vi "Unsubscribe Class Topic.vi"(7 "Close if last?":bool, 8 "error in (no error)":errorcluster, 10 "Receivers Enqueuer":refnum<class "Message Enqueuer.lvclass">, 11 "Topic":refnum<class>) -> (0 "error out":errorcluster)   [LabVIEW 2020, in "Actor Pub Sub Channels.lvlib"]
uses:
  Actor Pub Sub Channels.lvlib
  <vilib>/ActorFramework/Message Enqueuer/Message Enqueuer.lvclass
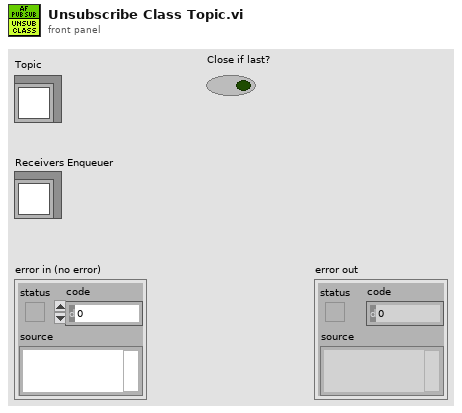
[diagram p1: front panel]
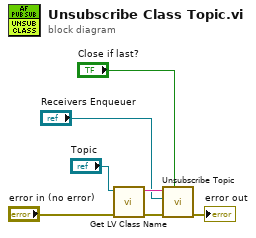
[diagram p0: block diagram]
diagram:
  n1 = call <vilib>:"Get LV Class Name.vi"("error in (no error)"="error in (no error)", "object"="Topic") -> ("error out"=w6:errorcluster, "class name"=w3:string)  [unwired: 8 in]
  n2 = call "Unsubscribe Topic.vi"("Close if last?"="Close if last?", "error in (no error)"=w6, "Receivers Enqueuer"="Receivers Enqueuer", "Topic  (ALL)"=w3) -> ("error out"=→"error out":errorcluster)  [unwired: 7 in]
